vi "Auton-Pickup.vi"(9 "Param 2":dbl=1.0, 10 "Param 1":dbl) -> (2 "Done":bool)   [LabVIEW 2014]
uses:
  Robot Global Data.vi
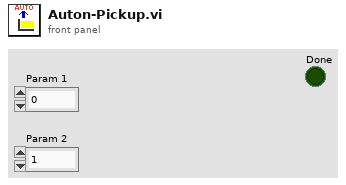
[diagram p1: front panel]
types:
  T1 = cluster{"Tote Constant":dbl, "Can2Catch Constant":dbl, "Bottom":dbl}
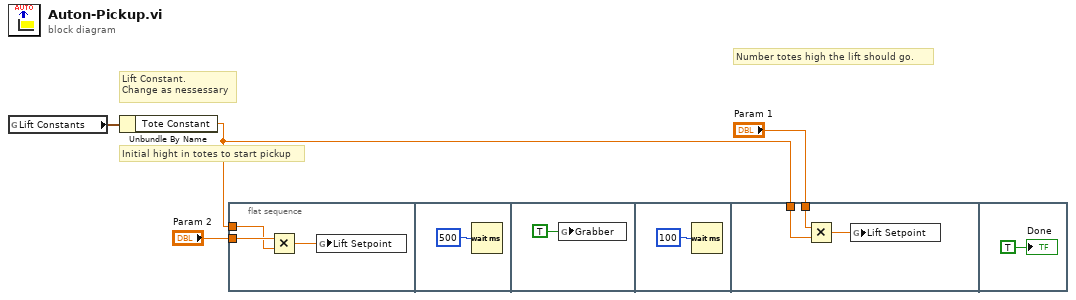
[diagram p0: block diagram]
diagram:
  # "Initial hight in totes to start pickup"
  # "Number totes high the lift should go."
  # "Lift Constant.\nChange as nessessary"
  n1 = global read "Robot Global Data.vi" "Lift Constants"() -> (w2:T1)
  n2 = Unbundle By Name(w2) -> ("Tote Constant"=w1:dbl)
  n3 = flat-sequence {
    tunnel: "Param 2" -> [w6]
    tunnel: w1 -> [w5]
    tunnel: "Param 1" -> [w13]
    tunnel: w1 -> [w11]
    frame #0 {
      n4 = Multiply(x=w6, y=w5) -> (x*y=w7:dbl)
      n5 = global write "Robot Global Data.vi" "Lift Setpoint"(w7) -> ()
    }
    frame #1 {
      n6 = Wait (ms)(milliseconds to wait=u32 500) -> ()  [unwired: 1 out]
    }
    frame #2 {
      n7 = global write "Robot Global Data.vi" "Grabber"(TRUE) -> ()
    }
    frame #3 {
      n8 = Wait (ms)(milliseconds to wait=u32 100) -> ()  [unwired: 1 out]
    }
    frame #4 {
      n9 = Multiply(x=w13, y=w11) -> (x*y=w12:dbl)
      n10 = global write "Robot Global Data.vi" "Lift Setpoint"(w12) -> ()
    }
    frame #5 {
      "Done" <- TRUE
    }
  }
